vi "refresh hardware dark corretion.vi"(8 "error in (no error)":errorcluster, 11 "LineCCD in":refnum<class "LineCCD.lvclass">) -> (0 "error out":errorcluster, 3 "LineCCD out":refnum<class "LineCCD.lvclass">)   [LabVIEW 2012, in "LineCCD.lvclass"]
uses:
  LineCCD.lvclass
  LineCCD.lvclass/LineCCD.ctl
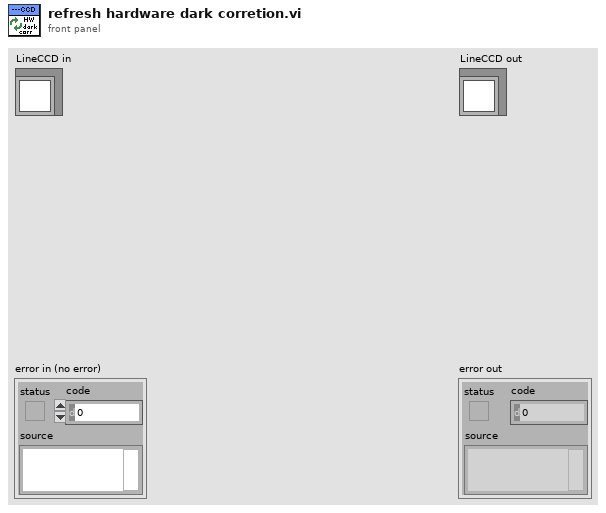
[diagram p1: front panel]
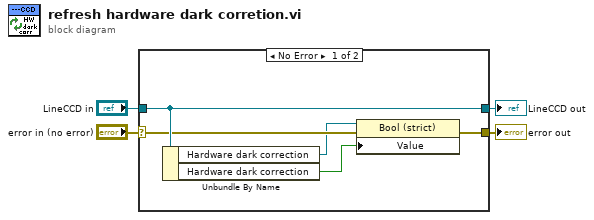
[diagram p0: block diagram]
diagram:
  n1 = case shown="No Error" "error in (no error)" {
    selector: "error in (no error)" -> [w8 w11]
    tunnel: [w7 w11] -> w3
    tunnel: [w9 w10] -> w1
    tunnel: "LineCCD in" -> [w9 w10]
    frame No Error {
      n2 = Unbundle By Name(w9) -> ("Hardware dark correction"=w6:refnum<vi>, "Hardware dark correction"=w5:bool)
      n3 = property class="Bool (strict)"(reference=w6, error in=w8, "Value"=w5) -> (error out=w7:errorcluster)  [unwired: 1 out]
    }
    frame Error {
    }
  }
  "error out" <- w3
  "LineCCD out" <- w1
